vi "lsl pull chunk d.vi"(0 "in":cluster{}, 1 "timestamp_buffer_elements":u32, 2 "ec":i32, 5 "data_buffer":dbl, 7 "timestamp_buffer":dbl, 9 "data_buffer_elements":u32, 11 "error in (no error)":errorcluster, 12 "timeout":dbl) -> (3 "function return":u32, 4 "in out":cluster{}, 6 "data_buffer out":dbl, 8 "timestamp_buffer out":dbl, 10 "ec out":i32, 15 "error out":errorcluster)   [LabVIEW 2018, in "liblsl-LabVIEW.lvlib"]
doc: "extern LIBLSL_C_API unsigned long lsl_pull_chunk_d(lsl_inlet in, double *data_buffer, double *timestamp_buffer, unsigned long data_buffer_elements, unsigned long timestamp_buffer_elements, double timeout, int32_t *ec);"
uses:
  <userlib>/liblsl-LabVIEW/liblsl-LabVIEW.lvlib
  <userlib>/liblsl-LabVIEW/liblsl64.dll
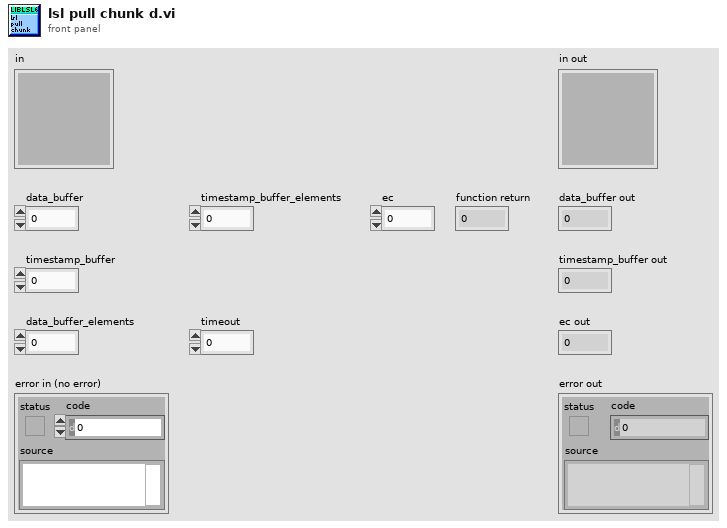
[diagram p1: front panel]
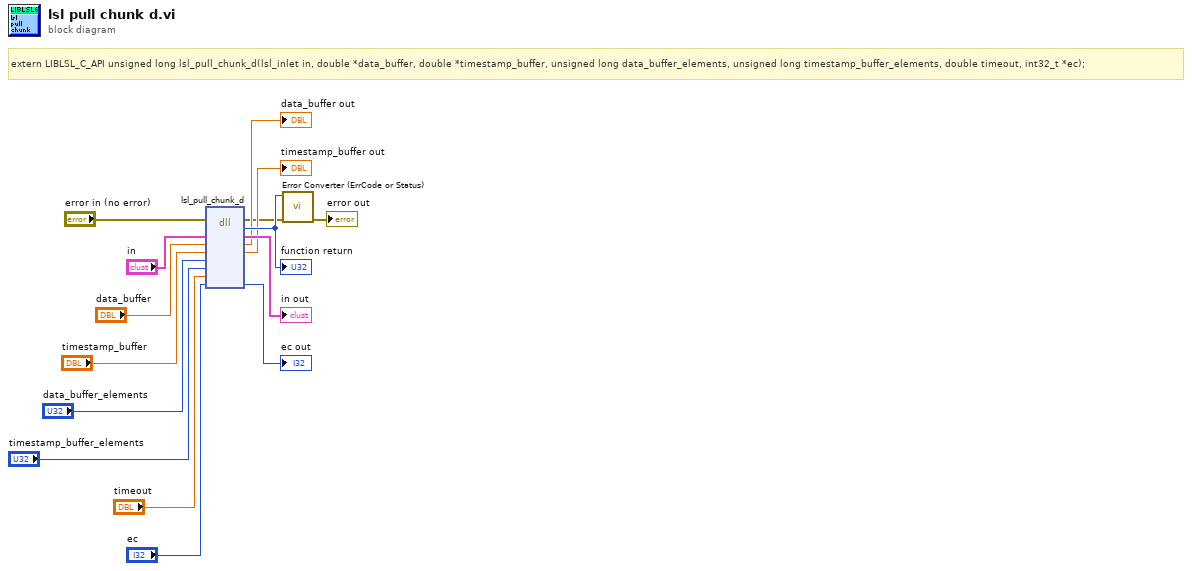
[diagram p0: block diagram]
diagram:
  # "extern LIBLSL_C_API unsigned long lsl_pull_chunk_d(lsl_inlet in, double *data_buffer, double *timestamp_buffer, unsigned long data_buffer_elements, unsigned long timestamp_buffer_elements, double timeout, int32_t *ec);"
  n1 = dll-call lib="C:/Program Files/National Instruments/LabVIEW 2018/user.lib/liblsl-LabVIEW/liblsl64.*" fn="lsl_pull_chunk_d"(error in="error in (no error)", "in"="in", "data_buffer"="data_buffer", "timestamp_buffer"="timestamp_buffer", "data_buffer_elements"="data_buffer_elements", "timestamp_buffer_elements"="timestamp_buffer_elements", "timeout"="timeout", "ec"="ec") -> (error out=w2:errorcluster, w15:u32, "in"=→"in out":cluster{}, "data_buffer"=→"data_buffer out":dbl, "timestamp_buffer"=→"timestamp_buffer out":dbl, "ec"=→"ec out":i32)  [unwired: 5 in, 1 out]
  "function return" <- w15
  n2 = call <userlib>:"Error Converter (ErrCode or Status).vi"("error in (no error)"=w2, "error code"=w15) -> ("error out"=→"error out":errorcluster)  [unwired: 9 in]
